vi "MallocMethod-NO-OPTMIZE.VI"(8 "error in (no error)":errorcluster) -> (0 "error out":errorcluster)   [LabVIEW 2017, in "MDPtr.lvlib" / "MDPtrMgr.lvclass"]
uses:
  MDPtrMgr.lvclass
  MDPtr TypeDef/MDPtr GlobalSettings.ctl
  MDPtr TypeDef/MDPtr MallocMethod.ctl
  MDPtr.lvlib
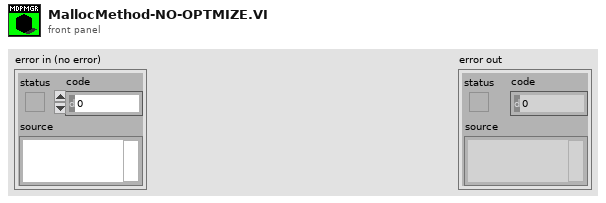
[diagram p1: front panel]
types:
  T1 = typedef "MDPtr.lvlib/MDPtr GlobalSettings.ctl" = cluster{"Malloc Method":T2, "FixedPreSize":cluster{"PreCacheSize":i32}}
  T2 = typedef "MDPtr.lvlib/MDPtr MallocMethod.ctl" = enum16{"NONE", "FIXED PRE-SIZE"}
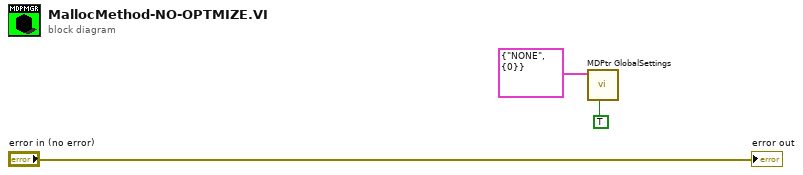
[diagram p0: block diagram]
diagram:
  n1 = call "MDPtr GlobalSettings.vi"("Oper(Get)"=TRUE, "Setting in"=T1 {"Malloc Method"=enum."NONE", "FixedPreSize"={"PreCacheSize"=0}}) -> ()  [unwired: 8 in, 2 out]
  "error out" <- "error in (no error)"
